vi "表格位置是否合法.vi"(8 "错误输入":errorcluster caption="错误输出", 10 "单元格位置":T1 caption="表格位置", 11 "引用输入":refnum<vi>) -> (0 "错误输出":errorcluster, 1 "是否在范围":bool, 2 "单元格位置输出":T1 caption="表格位置", 3 "引用输出":refnum<vi>)   [LabVIEW 2014, in "表格.lvlib"]
uses:
  <vilib>/Utility/miscctls.llb/LVRowAndColumnTypeDef.ctl
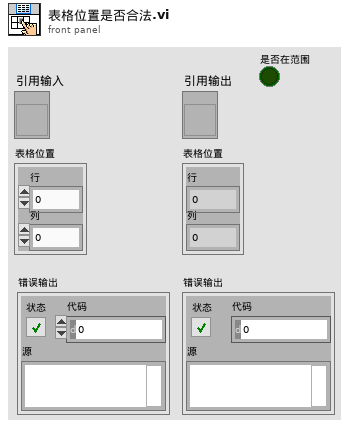
[diagram p1: front panel]
types:
  T1 = typedef "LVRowAndColumnTypeDef.ctl" = cluster{"Row":i32, "Column":i32}
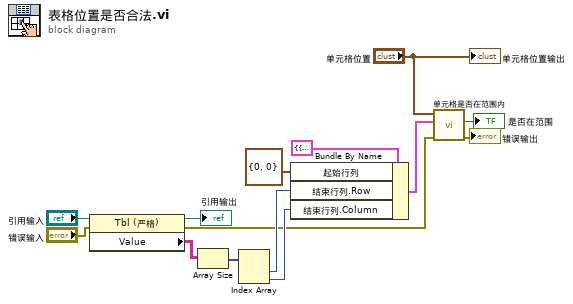
[diagram p0: block diagram]
diagram:
  n1 = property class="Tbl (严格)"(reference="引用输入", error in="错误输入") -> (reference out=→"引用输出":refnum<vi>, error out=w2:errorcluster, "Value"=w13:string[][])
  n2 = Array Size(array=w13) -> (size(s)=w9:i32[])
  n3 = Index Array(array=w9) -> (element #1=w8:i32, element #2=w7:i32)  [unwired: 2 in]
  n4 = Bundle By Name(cluster=cluster{"起始行列":T1, "结束行列":T1} {"起始行列"={"Row"=0, "Column"=0}, "结束行列"={"Row"=0, "Column"=0}} ("行列范围"), "起始行列"=T1 {"Row"=0, "Column"=0}, "结束行列.Row"=w8, "结束行列.Column"=w7) -> (w6:cluster{"起始行列":T1, "结束行列":T1})
  n5 = call "单元格是否在范围内.vi"("error in (no error)"=w2, "行列范围"=w6, "单元格位置"="单元格位置") -> ("error out"=→"错误输出":errorcluster, "是否在范围"=→"是否在范围":bool)  [unwired: 6 in, 1 out]
  "单元格位置输出" <- "单元格位置"
